vi "Target-Scoped FIFO (1xI16) - Read.vi"(2 "reset":bool, 11 "Target-Scoped FIFO (1xI16)":T2, 12 "ready for output (T)":bool=TRUE) -> (3 "reset done":bool, 4 "data out":T1, 6 "output valid":bool, 15 "elements to read":u32)   [LabVIEW 2018, in "Streaming FPGA.lvlib"]
doc: "Reads a Target-scoped FIFO using the data type provided by the <B>Data Type (1xI16).ctl</B>.\n\nSetting the <B>reset</B> input to true sets the <B>reset done</B> output to false and starts flushing any remaining samples from the FIFO. The reset cycle completes when the <B>reset out</B> output becomes true.\n\n<B>elements to read</B> is the number of elements that was available for reading in the FIFO in the previous clock cycle."
uses:
  Streaming FPGA.lvlib
  Target-Scoped FIFO (1xI16) Resource.ctl
  Data Type (1xI16).ctl
  <vilib>/rvi/DataTransferAndStorage/Container/Common/niFpgaContainerExecOnDevCompGetState.vi
  <vilib>/rvi/Emulation/niFpgaEmulationIsFPGAContextNoSignature.vi
  <vilib>/rvi/Emulation/niFpgaSctlEmulationGetInTimedLoop.vi
  <vilib>/rvi/errors/niFpgaSetErrorForExecOnDevCompSimple.vi
  <vilib>/rvi/eio/common/nirviEmuReportErrorAndStop.vi
  <vilib>/rvi/DataTransferAndStorage/Container/Common/niFpgaContainerGetUniqueNameForEmu.vi
  <vilib>/rvi/FIFO/Fifo_Resource/nirvififoEmulationSetSize.vi
  <vilib>/rvi/FIFO/Fifo_Resource/nirviFifoEmulationQueueMgr.vi
  <instcachedir>/0/nirviFifoEmulationQueueMgr_E5CAEC123FF24DC58D834DCA3CDAA9B5.lvgen/nirviFifoEmulationQueueMgr_E5CAEC123FF24DC58D834DCA3CDAA9B5_043.vi
  <vilib>/rvi/FIFO/Fifo_Resource/nirvififoEmulationDetermineInputValidOut.vi
  <vilib>/rvi/FIFO/Fifo_Resource/nirvififoEmulationCreateLock.vi
  <vilib>/rvi/Emulation/niFpgaProcessEmulError.vi
  <vilib>/rvi/FIFO/Fifo_Resource/nirvififoEmulationObtainLock.vi
  <vilib>/rvi/FIFO/Fifo_Resource/nirvififoEmulationReleaseLock.vi
  <vilib>/rvi/occurrence/nirviWaitOnOccurrenceBase.vi
  <vilib>/rvi/errors/nirviReportUnexpectedCaseInternalError.vi
  <vilib>/rvi/errors/nirviReportUnexpectedCaseInternalError (U32).vi
  <vilib>/Utility/error.llb/Clear Errors.vi
  <vilib>/rvi/interface/RandomDataEmulation/niFpgaRandomDataHandleErrors.vi
  <vilib>/rvi/DataTransferAndStorage/Container/XNode/niFpgaContainer.xnode
  <vilib>/rvi/FIFO/Fifo_Resource/niFpgaFifoEmulationRefIn.vi
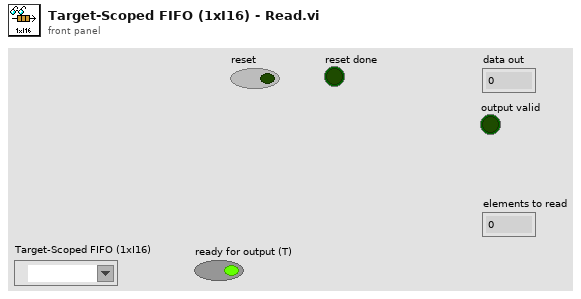
[diagram p1: front panel]
types:
  T1 = typedef "Streaming FPGA.lvlib/Data Type (1xI16).ctl" = i16
  T2 = typedef "Streaming FPGA.lvlib/Target-Scoped FIFO (1xI16) Resource.ctl" = refnum<k21>
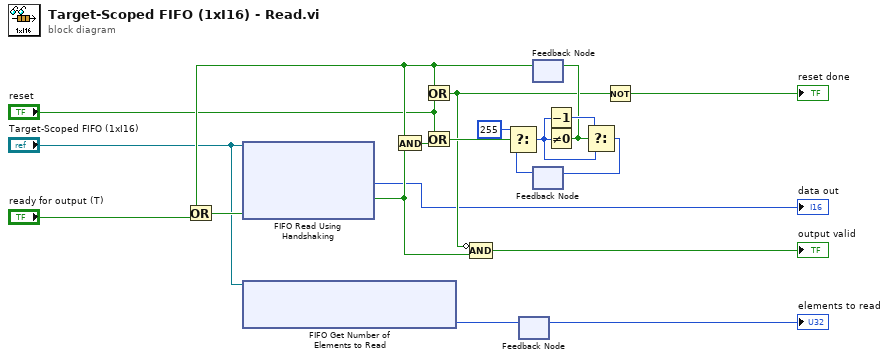
[diagram p0: block diagram]
diagram:
  n1 = xnode "FIFO Get Number of Elements to Read"("FIFO In"="Target-Scoped FIFO (1xI16)") -> ("Number of Elements to Read"=w3:u32)  [unwired: 1 out]
  n2 = feedback-in #1(w3) -> ()
  n3 = feedback #1() -> (→"elements to read":u32)  [unwired: 1 in]
  n4 = feedback #2() -> (w20:bool)  [unwired: 1 in]
  n5 = Or(x=w20, y="ready for output (T)") -> (x .or. y?=w8:bool)
  n6 = xnode "FIFO Read Using Handshaking"("Ready for Output"=w8, "FIFO In"="Target-Scoped FIFO (1xI16)") -> ("Element"=→"data out":i16, "Output Valid"=w7:bool)  [unwired: 1 out]
  n7 = And(x=w20, y=w7) -> (x .and. y?=w10:bool)
  n8 = Or(x=w20, y="reset") -> (x .or. y?=w6:bool)
  n9 = Or(x="reset", y=w10) -> (x .or. y?=w16:bool)
  n10 = Compound Arithmetic op=AND(invert w6, w7) -> (→"output valid":bool)
  n11 = feedback #3() -> (w12:u8)  [unwired: 1 in]
  n12 = Select(t=u8 255, s=w16, f=w12) -> (s? t:f=w15:u8)
  n13 = Decrement(x=w15) -> (x-1=w14:u8)
  n14 = Not Equal To 0?(x=w15) -> (x != 0?=w11:bool)
  n15 = feedback-in #2(w11) -> ()
  n16 = Select(t=w14, s=w11, f=w15) -> (s? t:f=w13:u8)
  n17 = feedback-in #3(w13) -> ()
  n18 = Not(x=w6) -> (.not. x?=→"reset done":bool)
